vi "Timer.vi"(7 "Cmd":enum16{"Reset", "Read"}(ring), 8 "error in (no error)":errorcluster) -> (0 "error out":errorcluster, 2 "Elapsed Time":dbl)   [LabVIEW 2009]
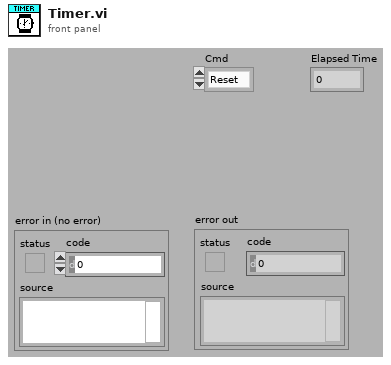
[diagram p1: front panel]
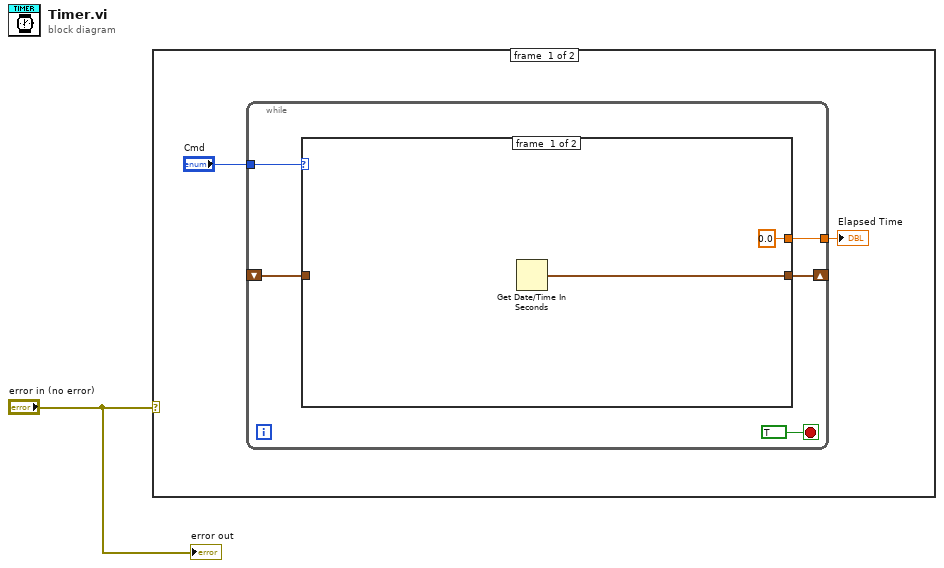
[diagram p0: block diagram]
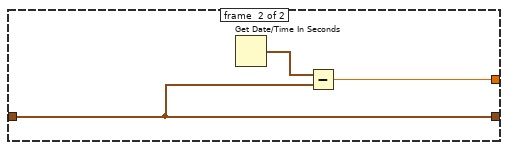
[diagram p2: hidden frame]
diagram:
  n1 = case shown="No Error" "error in (no error)" {
    frame #0 {
      n2 = while {
        tunnel: "Cmd" -> [w7]
        shift-right: [w6] -> _
        shift-left: _ -> [w5]
        tunnel: [w4] -> w2
        stop <- TRUE stop-if-true
        n3 = case shown="\"Read\"" w7 {
          tunnel: [w10 w12] -> w6
          tunnel: w5 -> [_ w12]
          tunnel: [0.0 w11] -> w4
          frame #0 {
            n4 = Get Date/Time In Seconds() -> (seconds since 1Jan1904=w10:timestamp)
          }
          frame #1 {
            n5 = Get Date/Time In Seconds() -> (seconds since 1Jan1904=w13:timestamp)
            n6 = Subtract(x=w13, y=w12) -> (x-y=w11:dbl)
          }
        }
      }
      "Elapsed Time" <- w2
    }
    frame #1 {
    }
  }
  "error out" <- "error in (no error)"
